vi "Test Database Tools.vi"() -> ()   [LabVIEW 2013]
doc: "This sub-VI tests using the database connectivity toolkit to save and data in a structured database."
uses:
  <vilib>/addons/database/Connection.llb/DB Tools Open Connec (String).vi
  <vilib>/addons/database/NI_Database_API.lvlib
panel:
  in  "connection information":string="mySQL measurement data"
  in  "Drop table?":bool
  in  "Result":string="Good"
  in  "Test number":dbl=1.0
  in  "Unit under test":string="unit 1"
  in  "columns":string[](array[string])=["Unit_under_test", "Test_number", "Result", "Array"]
  in  "table":string="unit_tests"
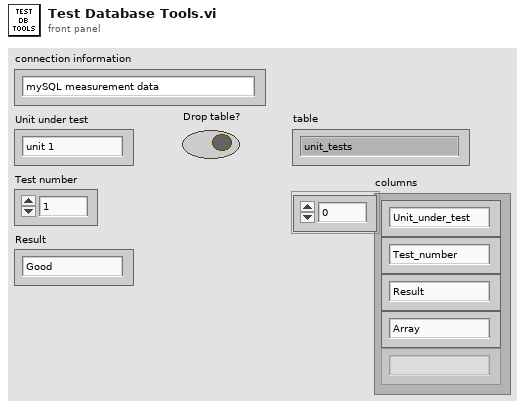
[diagram p1: front panel]
types:
  T1 = typedef "NI_Database_API.lvlib/Conn ObjectReference.ctl" = refnum<k1>
  T2 = cluster{"Unit under test":string, "Test number":dbl, "Result":string, "JSON string":string, "seconds since 1Jan1904":timestamp}
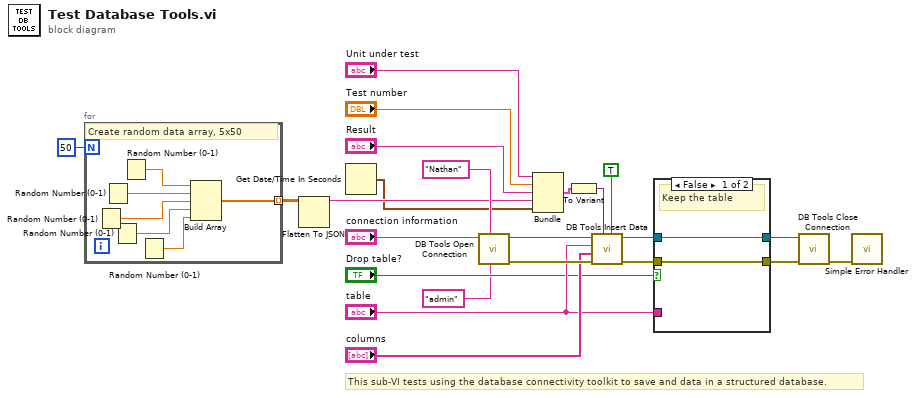
[diagram p0: block diagram]
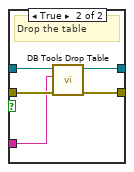
[diagram p2: hidden frame]
diagram:
  # "This sub-VI tests using the database connectivity toolkit to save and data in a structured database."
  n1 = for {
    N: 50 -> [_]
    tunnel: [w24] -> w2 mode=indexing
    # "Create random data array, 5x50"
    n2 = Random Number (0-1)() -> (number: 0 to 1=w27:dbl)
    n3 = Random Number (0-1)() -> (number: 0 to 1=w28:dbl)
    n4 = Random Number (0-1)() -> (number: 0 to 1=w25:dbl)
    n5 = Random Number (0-1)() -> (number: 0 to 1=w29:dbl)
    n6 = Random Number (0-1)() -> (number: 0 to 1=w26:dbl)
    n7 = Build Array(w29, w28, w27, w25, w26) -> (w24:dbl[])
  }
  n8 = Flatten To JSON(anything=w2) -> (JSON string=w4:string)  [unwired: 2 in, 1 out]
  n9 = Get Date/Time In Seconds() -> (seconds since 1Jan1904=w1:timestamp)
  n10 = call-poly <vilib>:"DB Tools Open Connection.vi"("password"="admin", "userID"="Nathan", "connection information"="connection information") -> ("error out"=w23:errorcluster, "connection reference"=w20:T1)  [unwired: 5 in]
  n11 = Bundle("Unit under test"="Unit under test", "Test number"="Test number", "Result"="Result", "JSON string"=w4, "seconds since 1Jan1904"=w1) -> (w21:T2)  [unwired: 1 in]
  n12 = To Variant(anything=w21) -> (Variant=w8:variant)
  n13 = call <vilib>:"DB Tools Insert Data.vi"("create table? (F)"=TRUE, "data"=w8, "error in (no error)"=w23, "columns"="columns", "table"="table", "connection reference"=w20) -> ("error out"=w14:errorcluster, "connection reference out"=w12:T1)  [unwired: 4 in]
  n14 = case shown="False" "Drop table?" {
    tunnel: w14 -> [w30 w36]
    tunnel: [w30 w35] -> w13
    tunnel: w12 -> [w31 w34]
    tunnel: [w31 w33] -> w11
    tunnel: "table" -> [_ w32]
    frame False {
      # "Keep the table"
    }
    frame True {
      # "Drop the table"
      n15 = call <vilib>:"DB Tools Drop Table.vi"("error in (no error)"=w36, "table"=w32, "connection reference"=w34) -> ("error out"=w35:errorcluster, "connection reference out"=w33:T1)  [unwired: 5 in]
    }
  }
  n16 = call <vilib>:"DB Tools Close Connection.vi"("error in (no error)"=w13, "connection reference"=w11) -> ("error out"=w19:errorcluster)  [unwired: 5 in]
  n17 = call <vilib>:"Simple Error Handler.vi"("error in (no error)"=w19) -> ()  [unwired: 4 in, 5 out]
